vi "BallPlacementReceiverRole.vi"(7 "first call":bool, 8 "error in (no error)":errorcluster, 9 "Tactic index in":i32, 10 "Game in":refnum<class "Game.lvclass">, 11 "BallPlacementReceiverRole in":refnum<class "BallPlacementReceiverRole.lvclass">) -> (0 "error out":errorcluster, 1 "tactic index out":i32, 2 "Robot out":refnum<class "Robot.lvclass">, 3 "BallPlacementReceiverRole out":refnum<class "BallPlacementReceiverRole.lvclass">)   [LabVIEW 2020, in "BallPlacementReceiverRole.lvclass"]
uses:
  BallPlacementReceiverRole.lvclass
  C:/RoboIME/SSL_AI/Role_class/Role.lvclass
  Game_class/Game.lvclass
  Robot_class/Robot.lvclass
  Role_class/Role.lvclass/Role.ctl
  BallPlacementReceiverRole.lvclass/BallPlacementReceiverRole.ctl
  Tacticbook_class/Tacticbook.lvclass/Tacticbook.ctl
  GoToBallPlacementPositionTactic_class/GoToBallPlacementPositionTactic.lvclass/GoToBallPlacementPositionTactic.ctl
  PlaceBallTactic_class/PlaceBallTactic.lvclass/PlaceBallTactic.ctl
  Tacticbook_class/Read GoToBallPlacementPositionTactic.vi
  GoToBallPlacementPositionTactic_class/Read States.vi
  Tacticbook_class/Write GoToBallPlacementPositionTactic.vi
  Tacticbook_class/Read WaitPassTactic.vi
  Tacticbook_class/Write WaitPassTactic.vi
  Tacticbook_class/Read PlaceBallTactic.vi
  PlaceBallTactic_class/Read States.vi
  Tacticbook_class/Write PlaceBallTactic.vi
  Role_class/Read Tacticbook.vi
  Read number_of_tactics.vi
  Role_class/Read RobotRef.vi
  Role_class/Write Tacticbook.vi
  Role_class/Write tactic_index.vi
  Tacticbook_class/Tacticbook.lvclass
  GoToBallPlacementPositionTactic_class/GoToBallPlacementPositionTactic.lvclass
  WaitPassTactic_class/WaitPassTactic.lvclass
  PlaceBallTactic_class/PlaceBallTactic.lvclass
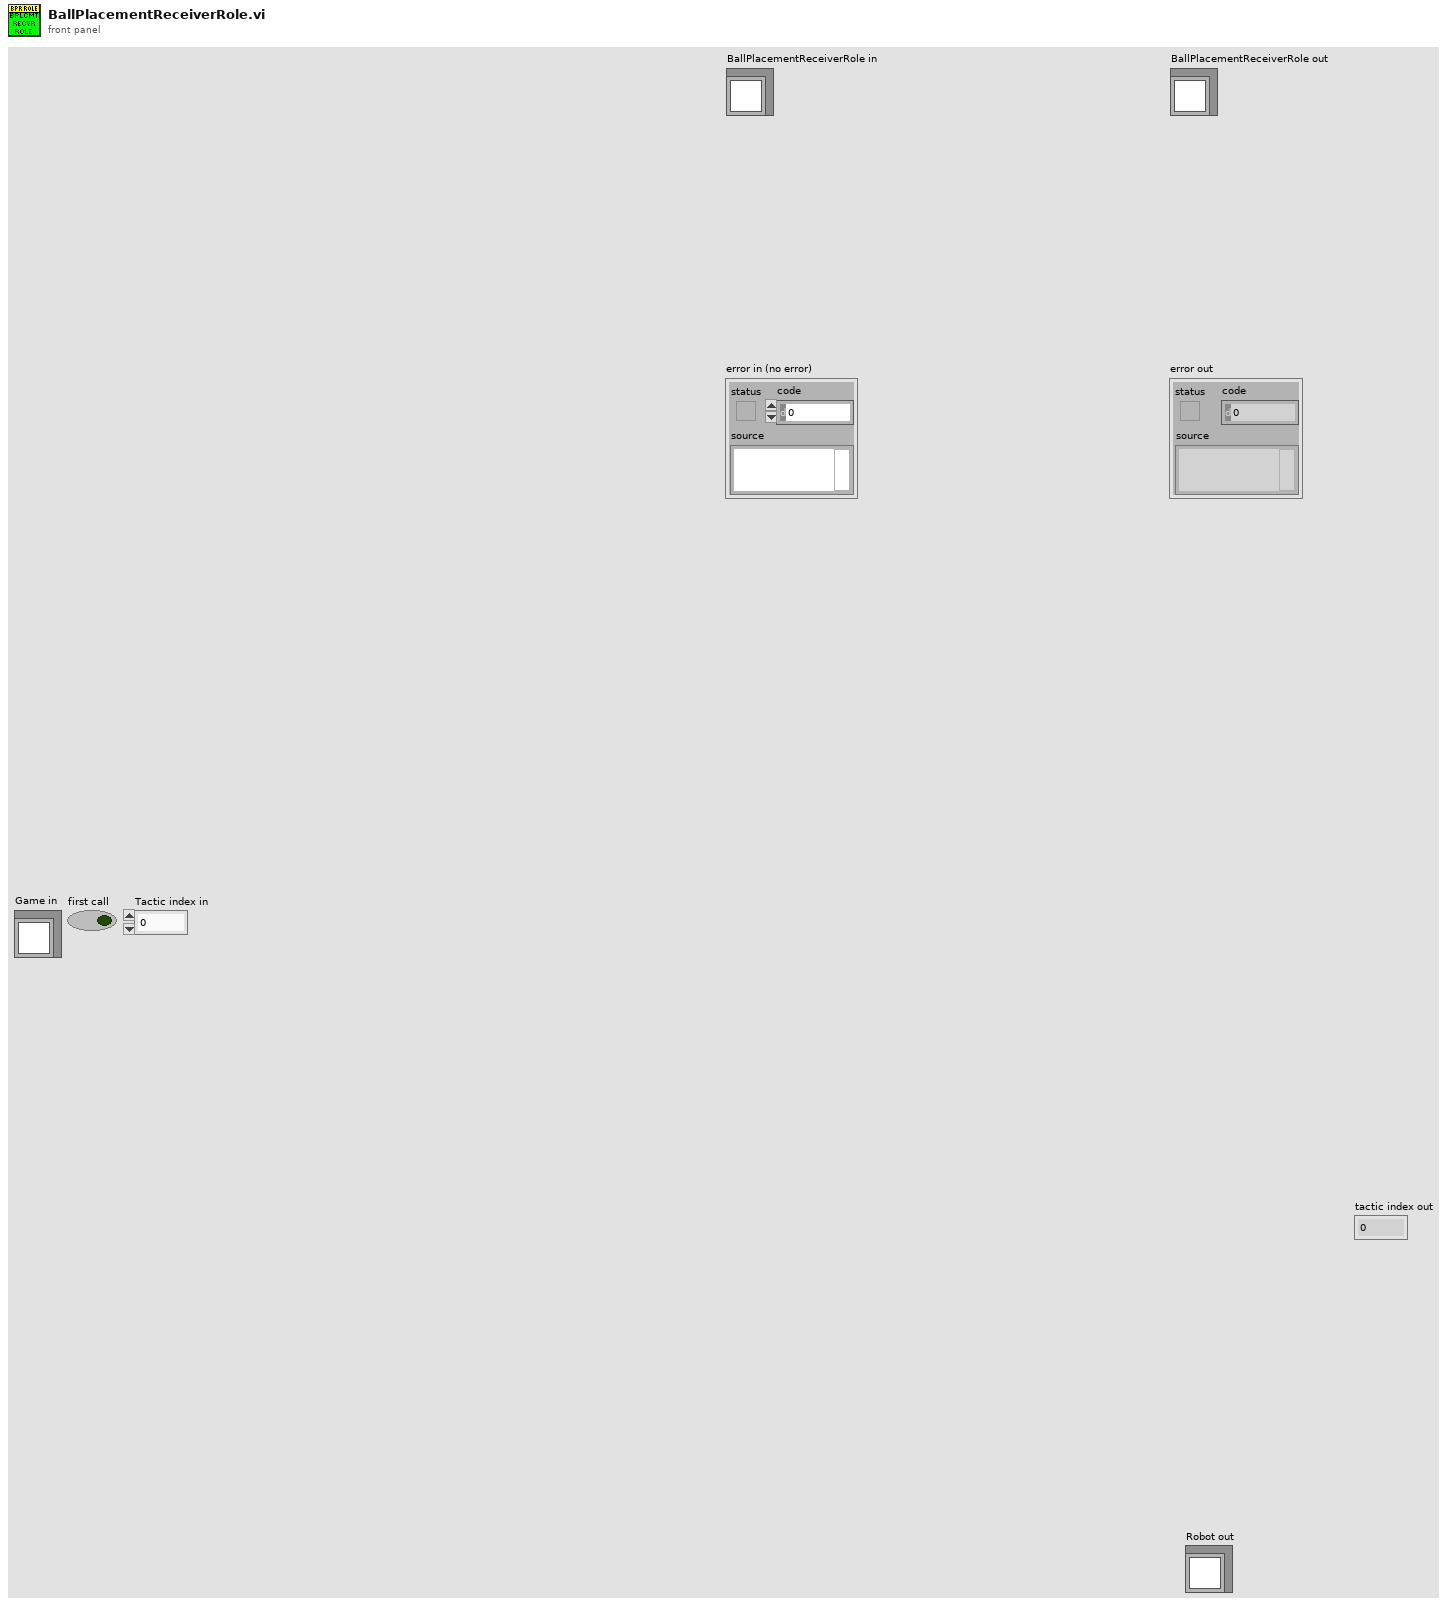
[diagram p1: front panel]
types:
  T1 = typedef "GoToBallPlacementPositionTactic.lvclass/StatesGoToBallPlacementPositionTactic.ctl" = enum16{"GoToPosition", "Exit"}
  T2 = typedef "StatesPlaceBallTactic.ctl" = enum16{"GoToGetBall", "PlaceBall", "Exit"}
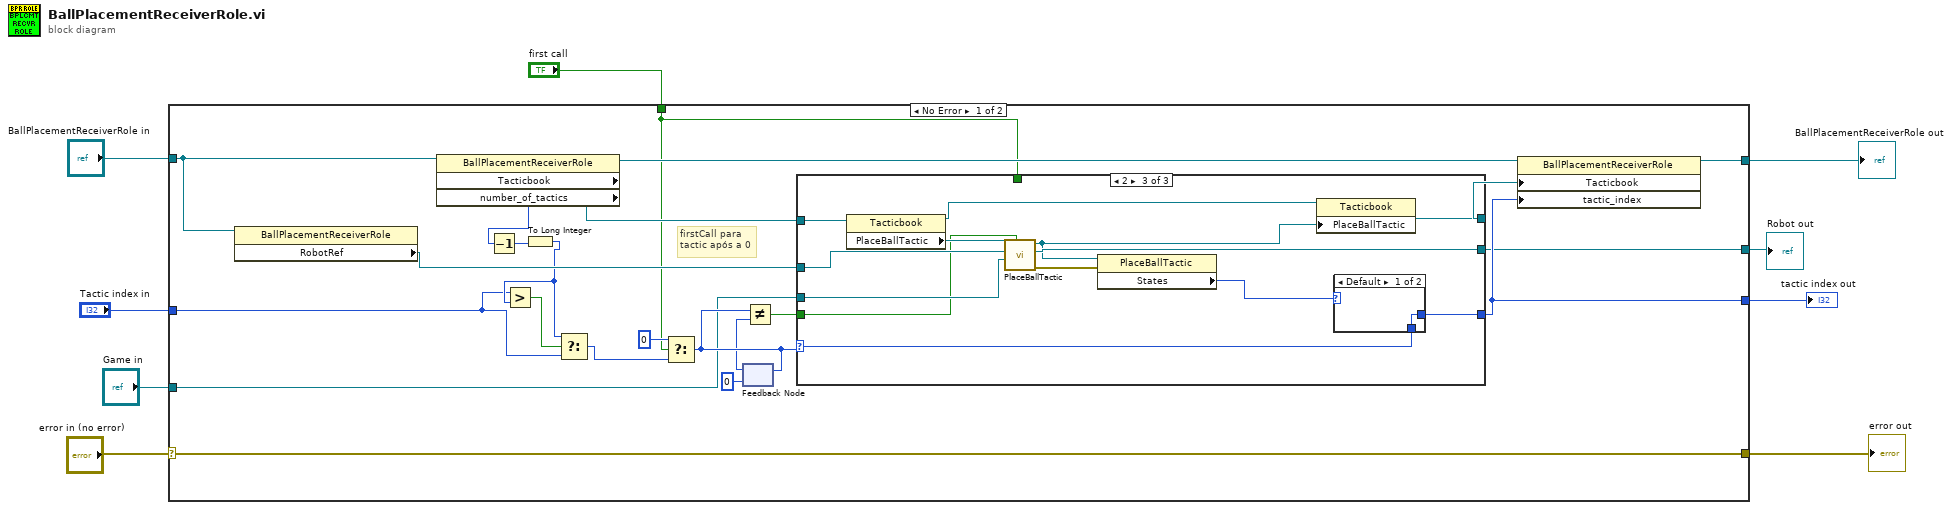
[diagram p0: block diagram]
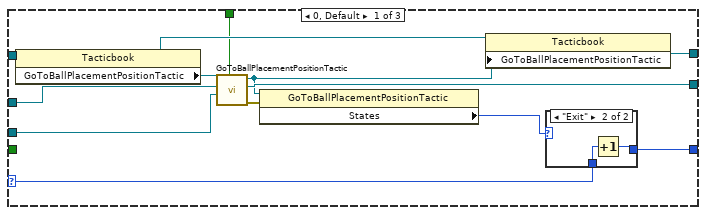
[diagram p2: hidden frame]
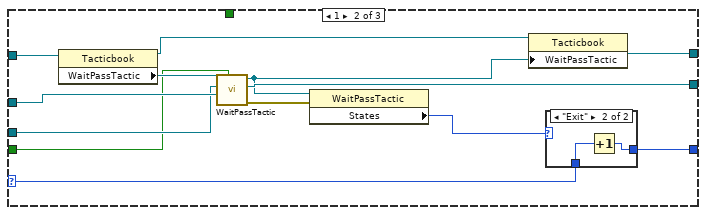
[diagram p4: hidden frame]
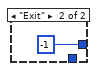
[diagram p6: hidden frame]
diagram:
  n1 = case shown="No Error" "error in (no error)" {
    selector: "error in (no error)" -> [w31 w80]
    tunnel: [w31 w80] -> w3
    tunnel: [w13 w79] -> w1
    tunnel: "BallPlacementReceiverRole in" -> [w16 w79]
    tunnel: "Tactic index in" -> [w15 _]
    tunnel: "Game in" -> [w14 _]
    tunnel: "first call" -> [w12 _]
    tunnel: [w11 _] -> w6
    tunnel: [w10 _] -> w5
    frame No Error {
      # "firstCall para\ntactic após a 0"
      n2 = property class="BallPlacementReceiverRole"(reference=w16) -> ("RobotRef"=w30:refnum<class "Robot.lvclass">)  [unwired: 1 in, 2 out]
      n3 = property class="BallPlacementReceiverRole"(reference=w16) -> (reference out=w29:refnum<class "BallPlacementReceiverRole.lvclass">, "Tacticbook"=w28:refnum<class "Tacticbook.lvclass">, "number_of_tactics"=w25:i32)  [unwired: 1 in, 1 out]
      n4 = Decrement(x=w25) -> (x-1=w24:i32)
      n5 = To Long Integer(number=w24) -> (32bit integer=w23:i32)
      n6 = Greater?(x=w15, y=w23) -> (0:w26:bool)
      n7 = Select(t=w23, s=w26, f=w15) -> (s? t:f=w22:i32)
      n8 = Select(t=0, s=w12, f=w22) -> (s? t:f=w20:i32)
      n9 = feedback #1(0 ("Tactic index in")) -> (w19:i32)
      n10 = feedback-in #1(w20) -> ()
      n11 = Not Equal?(x=w20, y=w19) -> (x != y?=w17:bool)
      n12 = case shown="2" w20 {
        selector: w20 -> [w33 w50 w66]
        tunnel: [w41 w57 w73] -> w11
        tunnel: w28 -> [w44 w60 w76]
        tunnel: w30 -> [w37 w54 w70]
        tunnel: [w42 w58 w74] -> w27
        tunnel: w14 -> [w36 w53 w69]
        tunnel: w12 -> [w39 _ _]
        tunnel: [w35 w52 w68] -> w10
        tunnel: w17 -> [_ w49 w65]
        frame 0, Default {
          n13 = property class="Tacticbook"(reference=w44) -> (reference out=w43:refnum<class "Tacticbook.lvclass">, "GoToBallPlacementPositionTactic"=w38:refnum<class "GoToBallPlacementPositionTactic.lvclass">)  [unwired: 1 in, 1 out]
          n14 = call "GoToBallPlacementPositionTactic.vi"("firstCall"=w39, "Game in"=w36, "Robot"=w37, "GoToBallPlacementPositionTactic in"=w38) -> ("error out"=w40:errorcluster, "Robot out"=w35:refnum<class "Robot.lvclass">, "GoToBallPlacementPositionTactic out"=w34:refnum<class "GoToBallPlacementPositionTactic.lvclass">)  [unwired: 5 in]
          n15 = property class="GoToBallPlacementPositionTactic"(reference=w34, error in=w40) -> ("States"=w32:T1)  [unwired: 2 out]
          n16 = property class="Tacticbook"(reference=w43, "GoToBallPlacementPositionTactic"=w34) -> (reference out=w42:refnum<class "Tacticbook.lvclass">)  [unwired: 1 in, 1 out]
          n17 = case shown="\"Exit\"" w32 {
            tunnel: [w45 w46] -> w41
            tunnel: w33 -> [w45 w47]
            frame Default {
            }
            frame "Exit" {
              n18 = Increment(x=w47) -> (x+1=w46:i32)
            }
          }
        }
        frame 1 {
          n19 = property class="Tacticbook"(reference=w60) -> (reference out=w59:refnum<class "Tacticbook.lvclass">, "WaitPassTactic"=w55:refnum<class "WaitPassTactic.lvclass">)  [unwired: 1 in, 1 out]
          n20 = call-dynamic "WaitPassTactic.vi"("first call"=w49, "Robot"=w54, "Game in"=w53, "WaitPassTactic in"=w55) -> ("error out"=w56:errorcluster, "Robot out"=w52:refnum<class "Robot.lvclass">, "WaitPassTactic out"=w51:refnum<class "WaitPassTactic.lvclass">)  [unwired: 5 in]
          n21 = property class="WaitPassTactic"(reference=w51, error in=w56) -> ("States"=w48:enum16{"State 0", "State 1", "State 2", "Exit"})  [unwired: 2 out]
          n22 = property class="Tacticbook"(reference=w59, "WaitPassTactic"=w51) -> (reference out=w58:refnum<class "Tacticbook.lvclass">)  [unwired: 1 in, 1 out]
          n23 = case shown="\"Exit\"" w48 {
            tunnel: [w61 w62] -> w57
            tunnel: w50 -> [w61 w63]
            frame Default {
            }
            frame "Exit" {
              n24 = Increment(x=w63) -> (x+1=w62:i32)
            }
          }
        }
        frame 2 {
          n25 = property class="Tacticbook"(reference=w76) -> (reference out=w75:refnum<class "Tacticbook.lvclass">, "PlaceBallTactic"=w71:refnum<class "PlaceBallTactic.lvclass">)  [unwired: 1 in, 1 out]
          n26 = call "PlaceBallTactic.vi"("firstCall"=w65, "Game in"=w69, "Robot"=w70, "PlaceBallTactic in"=w71) -> ("error out"=w72:errorcluster, "Robot out"=w68:refnum<class "Robot.lvclass">, "PlaceBallTactic out"=w67:refnum<class "PlaceBallTactic.lvclass">)  [unwired: 5 in]
          n27 = property class="PlaceBallTactic"(reference=w67, error in=w72) -> ("States"=w64:T2)  [unwired: 2 out]
          n28 = property class="Tacticbook"(reference=w75, "PlaceBallTactic"=w67) -> (reference out=w74:refnum<class "Tacticbook.lvclass">)  [unwired: 1 in, 1 out]
          n29 = case shown="Default" w64 {
            tunnel: [w77 -1] -> w73
            tunnel: w66 -> [w77 _]
            frame Default {
            }
            frame "Exit" {
            }
          }
        }
      }
      n30 = property class="BallPlacementReceiverRole"(reference=w29, "Tacticbook"=w27, "tactic_index"=w11) -> (reference out=w13:refnum<class "BallPlacementReceiverRole.lvclass">)  [unwired: 1 in, 1 out]
    }
    frame Error {
    }
  }
  "error out" <- w3
  "BallPlacementReceiverRole out" <- w1
  "Robot out" <- w5
  "tactic index out" <- w6
